vi "TPFL2dll.vi"(8 "error in (no error)":errorcluster, 11 "Inputs":T1) -> (0 "error out":errorcluster, 1 "herr_length":i32, 2 "herr":string, 3 "ierr":i32)   [LabVIEW 2016]
doc: "subroutine TPFL2dll(t, p, z, dl, dv, x, y, q, ierr, herr, herr_length)\n\nFlash calculation given temperature, pressure, and bulk composition. This routine accepts only two-phase states\nas inputs; if the phase is not known use TPFLSH. Use TPRHO for single-phase states.\n\nINPUTS: Two of the following\nt -- temperature [K]\np -- pressure [kPa]\nz -- overall (bulk) composition [array of mol frac]\nDl -- molar density [mol/L] of the liquid phase\nDv -- molar density [mol/L] of the vapor phase\nx -- composition of liquid phase [array of mol frac]\ny -- composition of vapor phase [array of mol frac]\nq -- vapor quality on a MOLAR basis [moles vapor/total moles]\n\nOUTPUTS:\n\nierr -- Error flag: (these are also passed up to TPFLSH for output) 0 - Successful\n 213 - TPRHO did not converge 226 - Iteration did not converge\nherr -- error string (character*255 variable if ierr<>0)\nherr_length -- length of variable herr (default: 255)"
uses:
  REFPROP.DLL
panel:
  # "REFPROP-TPFL2dll.vi"
  # "void  TPFL2dll(double *t, double *p, double *z, double *Dl, double *Dv, double *x, double *y, double *q, int32_t *ierr, CStr herr, int32_t herr_length)"
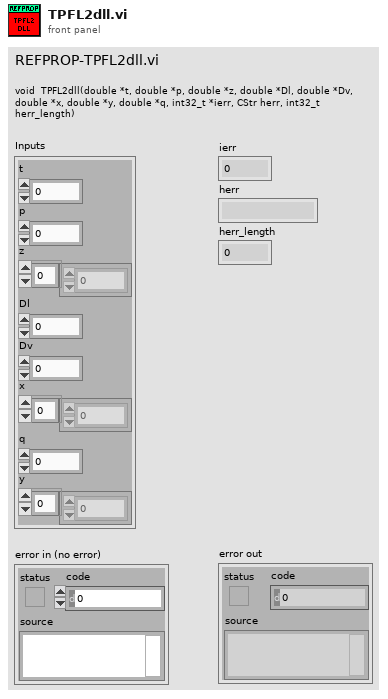
[diagram p1: front panel]
types:
  T1 = cluster{"t":dbl, "p":dbl, "z":dbl[], "Dl":dbl, "Dv":dbl, "x":dbl[], "y":dbl[], "q":dbl}
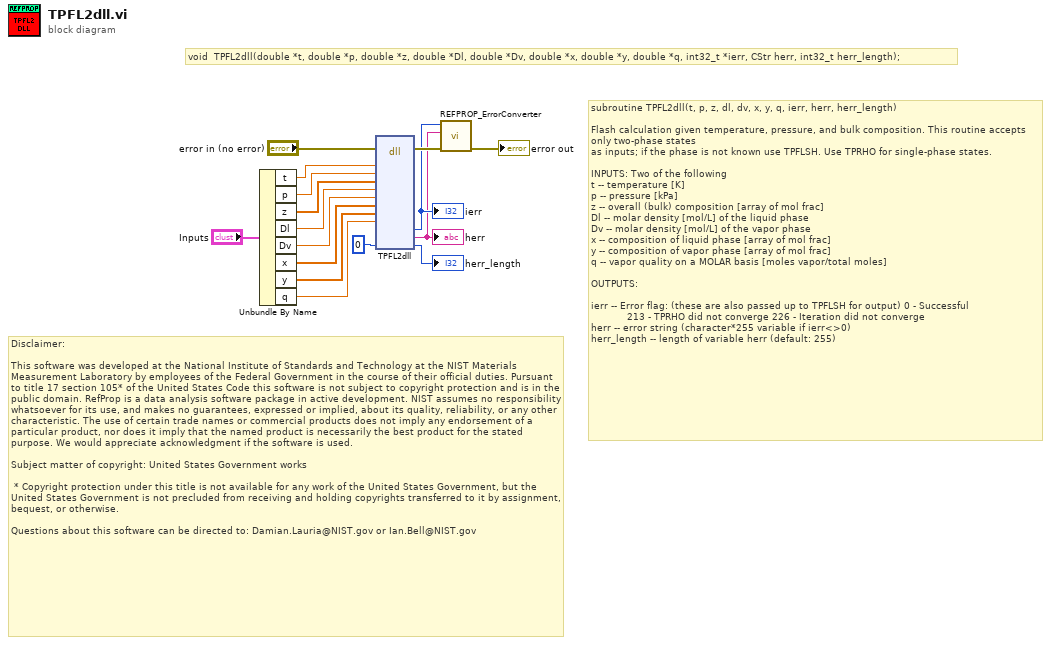
[diagram p0: block diagram]
diagram:
  # "Disclaimer:\n\nThis software was developed at the National Institute of Standards and Technology at the NIST Materials Measurement Laboratory by employees of the Federal Government in the course of their official duties. Pursuant to title 17 section 105* of the United States Code this software is not subject to copyright protection and is in the public domain. RefProp is a data analysis software package in active development. NIST assumes no responsibility whatsoever for its use, and makes no guarantees, expressed or implied, about its quality, reliability, or any other characteristic. The use of certain trade names or commercial products does not imply any endorsement of a particular product, nor does it imply that the named product is necessarily the best product for the stated purpose. We would appreciate acknowledgment if the software is used.\n \nSubject matter of copyright: United States Government works\n  \n * Copyright protection under this title is not available for any work of the United States Government, but the United States Government is not precluded from receiving and holding copyrights transferred to it by assignment, bequest, or otherwise.\n\nQuestions about this software can be directed to: Damian.Lauria@NIST.gov or Ian.Bell@NIST.gov"
  # "void  TPFL2dll(double *t, double *p, double *z, double *Dl, double *Dv, double *x, double *y, double *q, int32_t *ierr, CStr herr, int32_t herr_length);"
  # "subroutine TPFL2dll(t, p, z, dl, dv, x, y, q, ierr, herr, herr_length)\n\nFlash calculation given temperature, pressure, and bulk composition. This routine accepts only two-phase states\nas inputs; if the phase is not known use TPFLSH. Use TPRHO for single-phase states.\n\nINPUTS: Two of the following\nt -- temperature [K]\np -- pressure [kPa]\nz -- overall (bulk) composition [array of mol frac]\nDl -- molar density [mol/L] of the liquid phase\nDv -- molar density [mol/L] of the vapor phase\nx -- composition of liquid phase [array of mol frac]\ny -- composition of vapor phase [array of mol frac]\nq -- vapor quality on a MOLAR basis [moles vapor/total moles]\n\nOUTPUTS:\n\nierr -- Error flag: (these are also passed up to TPFLSH for output) 0 - Successful\n            213 - TPRHO did not converge 226 - Iteration did not converge\nherr -- error string (character*255 variable if ierr<>0)\nherr_length -- length of variable herr (default: 255)"
  n1 = Unbundle By Name("Inputs") -> ("t"=w8:dbl, "p"=w7:dbl, "z"=w6:dbl[], "Dl"=w5:dbl, "Dv"=w4:dbl, "x"=w3:dbl[], "y"=w2:dbl[], "q"=w1:dbl)
  n2 = dll-call lib="C:/Program Files (x86)/REFPROP/REFPROP.*" fn="TPFL2dll"(error in="error in (no error)", "t"=w8, "p"=w7, "z"=w6, "Dl"=w5, "Dv"=w4, "x"=w3, "y"=w2, "q"=w1, "herr_length"=0 ("ln")) -> (error out=w14:errorcluster, "ierr"=w12:i32, "herr"=w11:string, "herr_length"=→"herr_length":i32)  [unwired: 13 in, 1 out]
  "ierr" <- w12
  "herr" <- w11
  n3 = call "REFPROP_ErrorConverter.vi"("error in (no error)"=w14, "Error Message"=w11, "Error Code"=w12) -> ("error out"=→"error out":errorcluster)  [unwired: 8 in]
